vi "Has Active Nested.vi"(8 "error in (no error)":errorcluster, 11 "Module in":refnum<class "Module.lvclass">) -> (0 "error out":errorcluster, 2 "Has Active Nested":bool, 3 "Module out":refnum<class "Module.lvclass">)   [LabVIEW 2020, in "Volatus.lvlib" / "Module.lvclass"]
uses:
  Module.lvclass
  Module.lvclass/Module.ctl
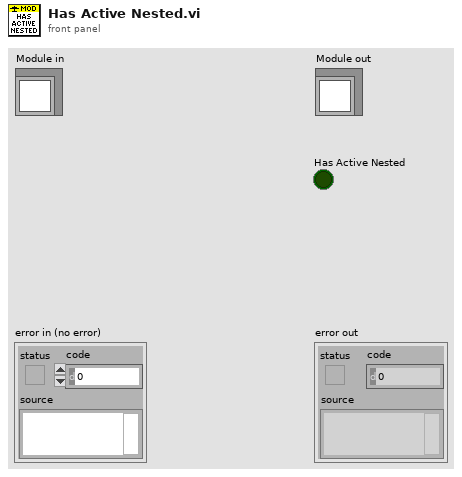
[diagram p1: front panel]
types:
  T1 = typedef "Volatus.lvlib/Module Status.ctl" = cluster{"MessageQ":refnum<class "MessageQ.lvclass">, "State":T2, "Hierarchy":string[], "Forwarded":bool}
  T2 = typedef "Volatus.lvlib/Module.lvclass/State.ctl" = enum16{"Unknown", "Launched", "Starting", "Running", "Stopping", "Stopped", "Error - Starting", "Error - Run", "Error - Stopping"}
  T3 = cluster{"MsgQ":refnum<class "MessageQ.lvclass">, "Status":T1}[]
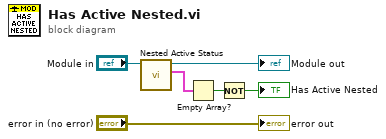
[diagram p0: block diagram]
diagram:
  n1 = call "Nested Active Status.vi"("Module in"="Module in") -> ("Active Nested"=w3:T3, "Module out"=→"Module out":refnum<class "Module.lvclass">)  [unwired: 7 in, 2 out]
  n2 = Empty Array?(array=w3) -> (empty?=w2:bool)
  n3 = Not(x=w2) -> (.not. x?=→"Has Active Nested":bool)
  "error out" <- "error in (no error)"
